vi "JAPCexitALLtypes.vi"(3 "Object out":refnum<class "JSubscribe.lvclass">, 8 "error in (no error)":errorcluster, 10 "Data Type":string) -> (0 "error out":errorcluster)   [LabVIEW 2014]
uses:
  <userlib>/_RADE/RIO/JAPC/classes/JSubscribe/openJAPCSubscribe.vi
  <userlib>/_RADE/RIO/JAPC/classes/JSubscribe/JSubscribe.lvclass
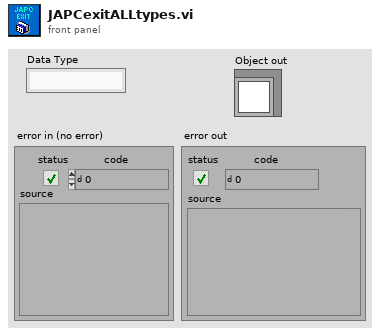
[diagram p1: front panel]
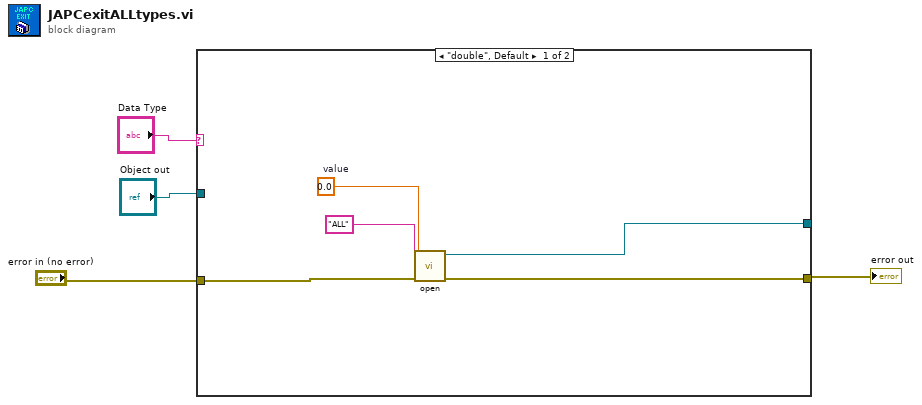
[diagram p0: block diagram]
diagram:
  n1 = case shown="\"double\", Default" "Data Type" {
    tunnel: "error in (no error)" -> [w6 w10]
    tunnel: [w7 w10] -> w2
    tunnel: [w5 _] -> _
    tunnel: "Object out" -> [_ _]
    frame "double", Default {
      w8 = 0.0  # value
      n2 = call-poly <userlib>:"open.vi"("error in (no error)"=w6, "Data type"=w8, "Cycle"="ALL") -> ("error out"=w7:errorcluster, "Object out"=w5:refnum<class "JSubscribe.lvclass">)  [unwired: 7 in]
    }
    frame "short" {
    }
  }
  "error out" <- w2
